vi "standard_angle.vi"(1 "angle in":dbl) -> (0 "angle out":dbl)   [LabVIEW 2023]
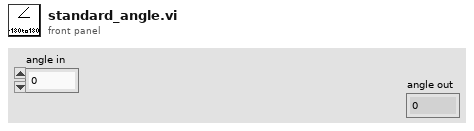
[diagram p1: front panel]
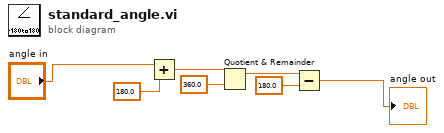
[diagram p0: block diagram]
diagram:
  n1 = Add(x="angle in", y=180.0) -> (x+y=w6:dbl)
  n2 = Quotient & Remainder(x=w6, y=360.0) -> (x-y*floor(x/y)=w4:dbl)  [unwired: 1 out]
  n3 = Subtract(x=w4, y=180.0) -> (x-y=→"angle out":dbl)
